vi "TCP Buffered Write.vi"(0 "connection ID":refnum<k5>, 5 "data string":string, 7 "packet size (bytes)":i32=32768, 9 "timeout (ms)":i32=5000, 11 "error in (no error)":errorcluster) -> (4 "connection ID 2":refnum<k5>, 8 "bytes written":i32, 15 "error out":errorcluster)   [LabVIEW 2015]
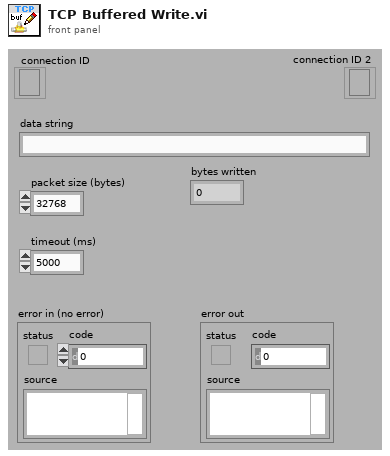
[diagram p1: front panel]
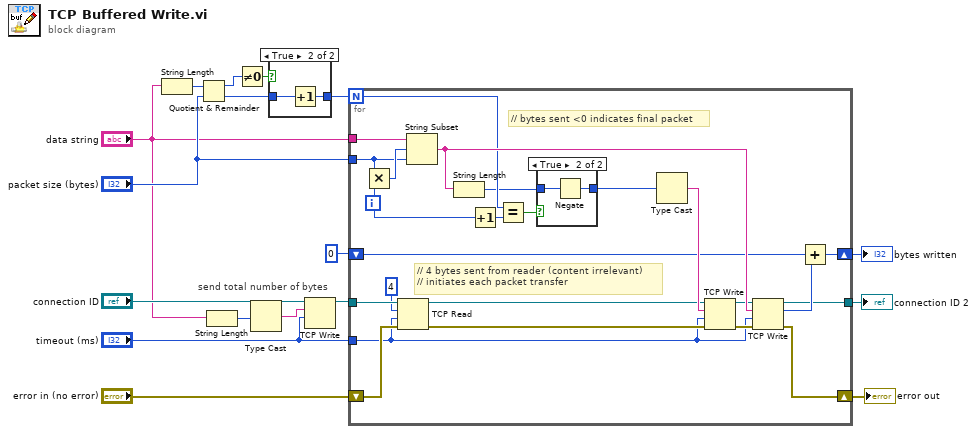
[diagram p0: block diagram]
diagram:
  # "send total number of bytes"
  n1 = String Length(string="data string") -> (length=w16:i32)
  n2 = Quotient & Remainder(x=w16, y="packet size (bytes)") -> (x-y*floor(x/y)=w15:i32, floor(x/y)=w12:i32)
  n3 = String Length(string="data string") -> (length=w1:i32)
  n4 = Not Equal To 0?(x=w15) -> (x != 0?=w13:bool)
  n5 = Type Cast(x=w1) -> (*(type *) &x=w4:string)  [unwired: 1 in]
  n6 = case shown="True" w13 {
    tunnel: w12 -> [w18 w20]
    tunnel: [w18 w19] -> w11
    frame False {
    }
    frame True {
      n7 = Increment(x=w20) -> (x+1=w19:i32)
    }
  }
  n8 = TCP Write(connection ID="connection ID", data in=w4, 9:"timeout (ms)") -> (connection ID out=w5:refnum<k5>)  [unwired: 1 in, 2 out]
  n9 = for {
    N: w11 -> [w29]
    tunnel: w5 -> [w36]
    shift-right: [w44] -> w17
    shift-left: "error in (no error)" -> [w35]
    tunnel: "data string" -> [w43]
    tunnel: "packet size (bytes)" -> [w41]
    tunnel: "timeout (ms)" -> [w32]
    shift-right: [w24] -> w8
    shift-left: 0 -> [w22]
    tunnel: [w21] -> w7
    i -> [w30]
    # "// bytes sent <0 indicates final packet"
    # "// 4 bytes sent from reader (content irrelevant)\n// initiates each packet transfer"
    n10 = Multiply(x=w41, y=w30) -> (x*y=w42:i32)
    n11 = TCP Read(connection ID=w36, bytes to read=4, error in (no error)=w35, 9:w32) -> (connection ID out=w34:refnum<k5>, error out=w33:errorcluster)  [unwired: 1 in, 1 out]
    n12 = String Subset(string=w43, offset (0)=w42, length (rest)=w41) -> (substring=w40:string)
    n13 = String Length(string=w40) -> (length=w26:i32)
    n14 = Increment(x=w30) -> (x+1=w28:i32)
    n15 = Equal?(x=w29, y=w28) -> (x = y?=w27:bool)
    n16 = case shown="True" w27 {
      tunnel: w26 -> [w45 w47]
      tunnel: [w45 w46] -> w25
      frame False {
      }
      frame True {
        n17 = Negate(x=w47) -> (-x=w46:i32)
      }
    }
    n18 = Type Cast(x=w25) -> (*(type *) &x=w39:string)  [unwired: 1 in]
    n19 = TCP Write(connection ID=w34, data in=w39, error in (no error)=w33, 9:w32) -> (connection ID out=w38:refnum<k5>, error out=w37:errorcluster)  [unwired: 1 out]
    n20 = TCP Write(connection ID=w38, data in=w40, error in (no error)=w37, 9:w32) -> (connection ID out=w21:refnum<k5>, bytes written=w23:i32, error out=w44:errorcluster)
    n21 = Add(x=w22, y=w23) -> (x+y=w24:i32)
  }
  "error out" <- w17
  "bytes written" <- w8
  "connection ID 2" <- w7
